vi "Distributor - Usr Ev Engine.vi"(8 "error in (no error)":errorcluster, 11 "Action":T3=enum."Get Refs") -> (0 "error out":errorcluster, 1 "Events Array":string[](array[string]), 2 "Usr Ev Refs":T2, 3 "Usr Ev Reg - Refs - cluster":T1)   [LabVIEW 2023, in "Actor_Message_Distributor.lvlib" / "Message_Distributor_Class.lvclass"]
uses:
  Message_Distributor_Class.lvclass
  Distributor - Ctrl - Action.ctl
  Distributor - Ctrl - Usr Ev Ref.ctl
  Distributor - Ctrl - Usr Ev Reg - Refs.ctl
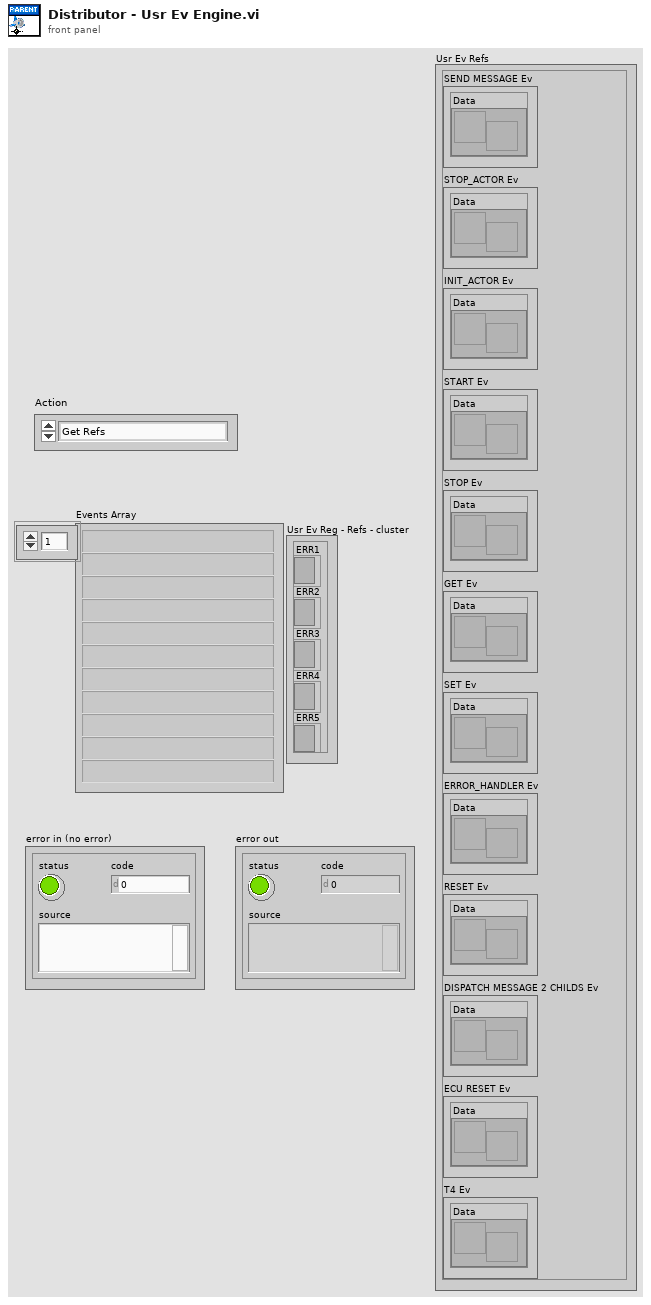
[diagram p1: front panel]
types:
  T1 = typedef "Actor_Message_Distributor.lvlib/Message_Distributor_Class.lvclass/Distributor - Ctrl - Usr Ev Reg - Refs.ctl" = cluster{"ERR1":refnum<event-registration>, "ERR2":refnum<event-registration>, "ERR3":refnum<event-registration>, "ERR4":refnum<event-registration>, "ERR5":refnum<event-registration>}
  T2 = typedef "Actor_Message_Distributor.lvlib/Message_Distributor_Class.lvclass/Distributor - Ctrl - Usr Ev Ref.ctl" = cluster{"SEND MESSAGE Ev":cluster{"Data":refnum<user-event>}, "STOP_ACTOR Ev":cluster{"Data":refnum<user-event>}, "INIT_ACTOR Ev":cluster{"Data":refnum<user-event>}, "START Ev":cluster{"Data":refnum<user-event>}, "STOP Ev":cluster{"Data":refnum<user-event>}, "GET Ev":cluster{"Data":refnum<user-event>}, "SET Ev":cluster{"Data":refnum<user-event>}, "ERROR_HANDLER Ev":cluster{"Data":refnum<user-event>}, "RESET Ev":cluster{"Data":refnum<user-event>}, "DISPATCH MESSAGE 2 CHILDS Ev":cluster{"Data":refnum<user-event>}, "ECU RESET Ev":cluster{"Data":refnum<user-event>}, "T4 Ev":cluster{"Data":refnum<user-event>}}
  T3 = typedef "Actor_Message_Distributor.lvlib/Message_Distributor_Class.lvclass/Distributor - Ctrl - Action.ctl" = enum16{"Reg Ev", "Get Refs", "Close Ev", "Populate Enum with Events"}
  T4 = enum32{"Invalid", "Standard", "Closed", "Hidden", "Minimized", "Maximized"}
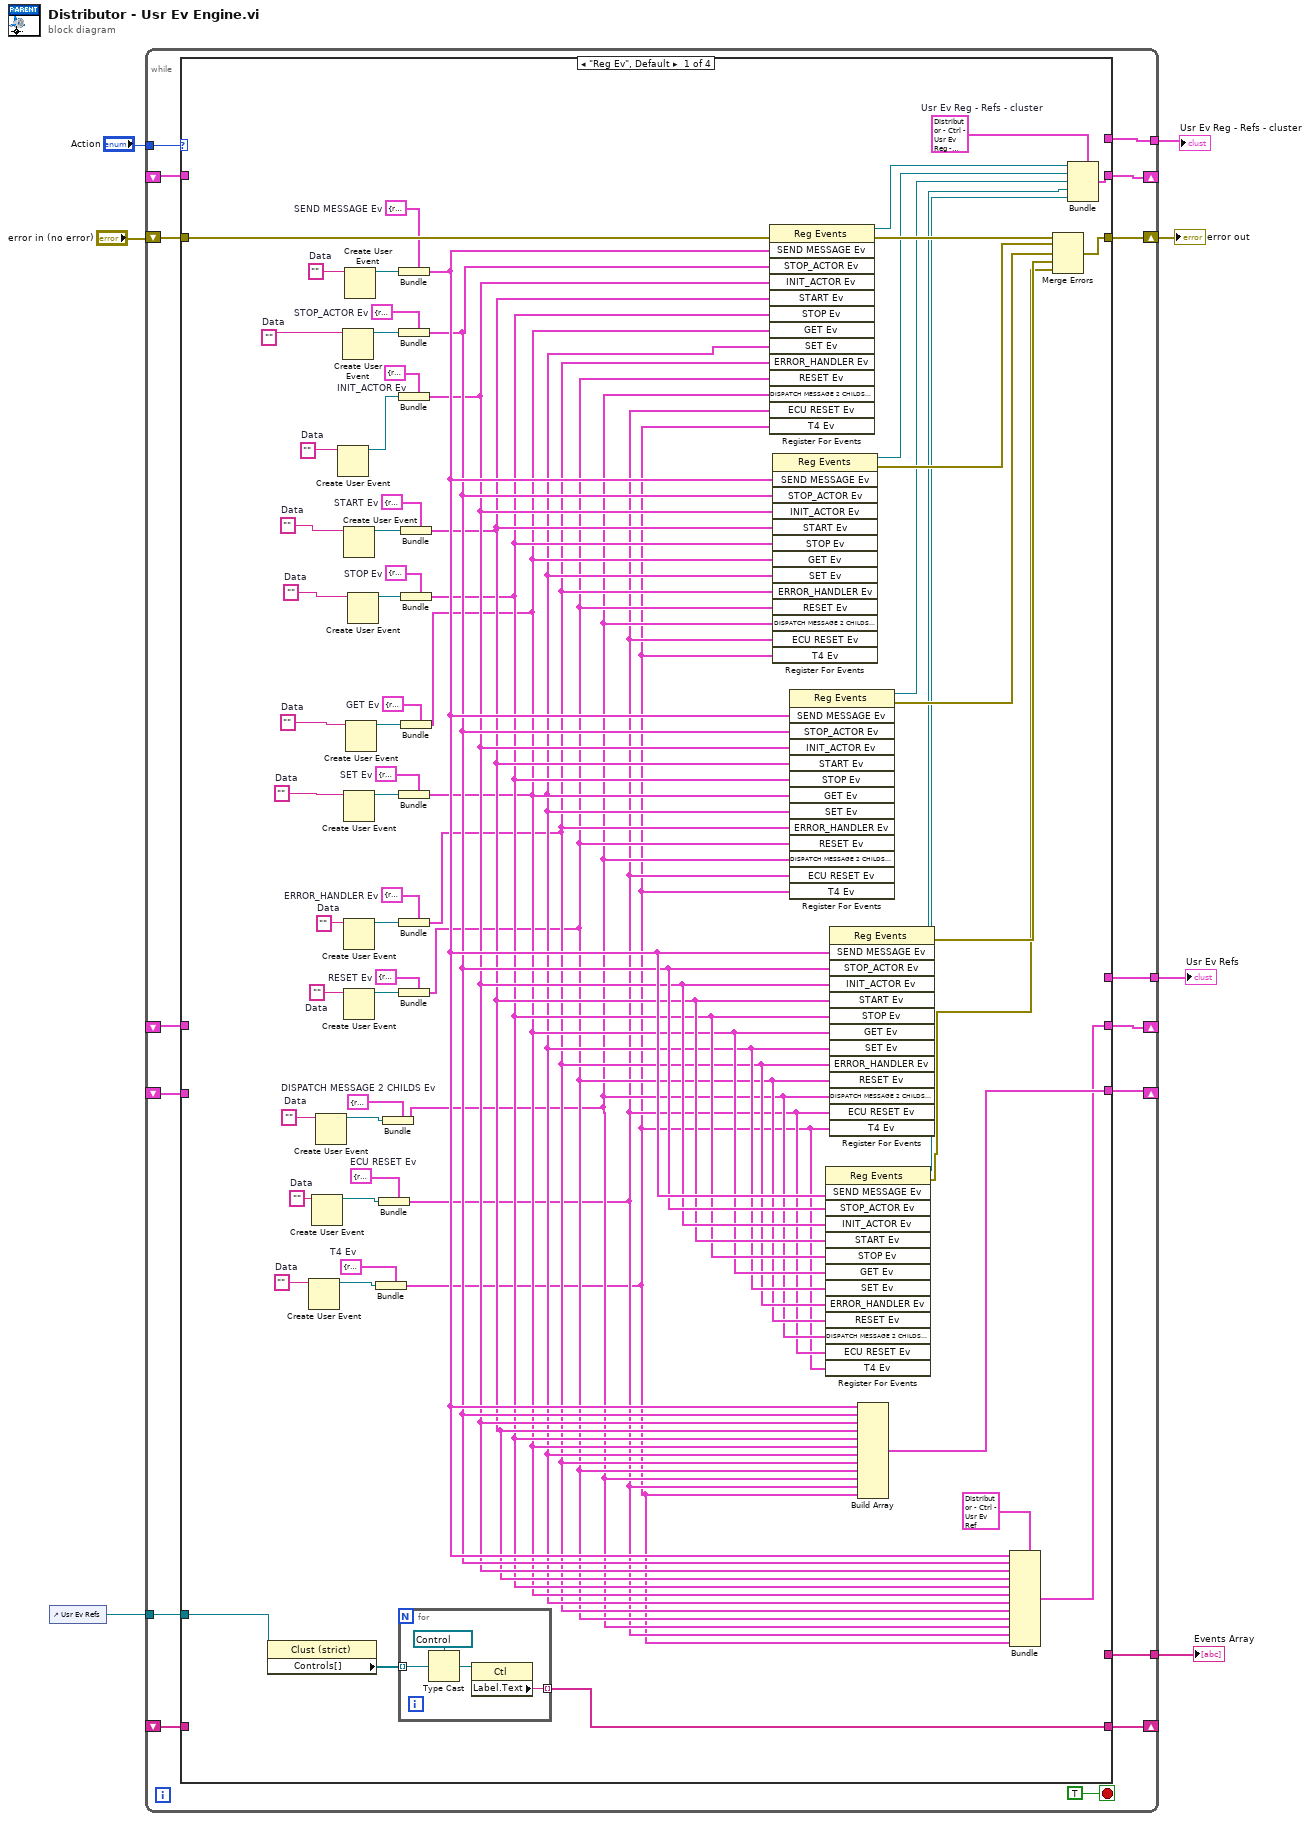
[diagram p0: block diagram]
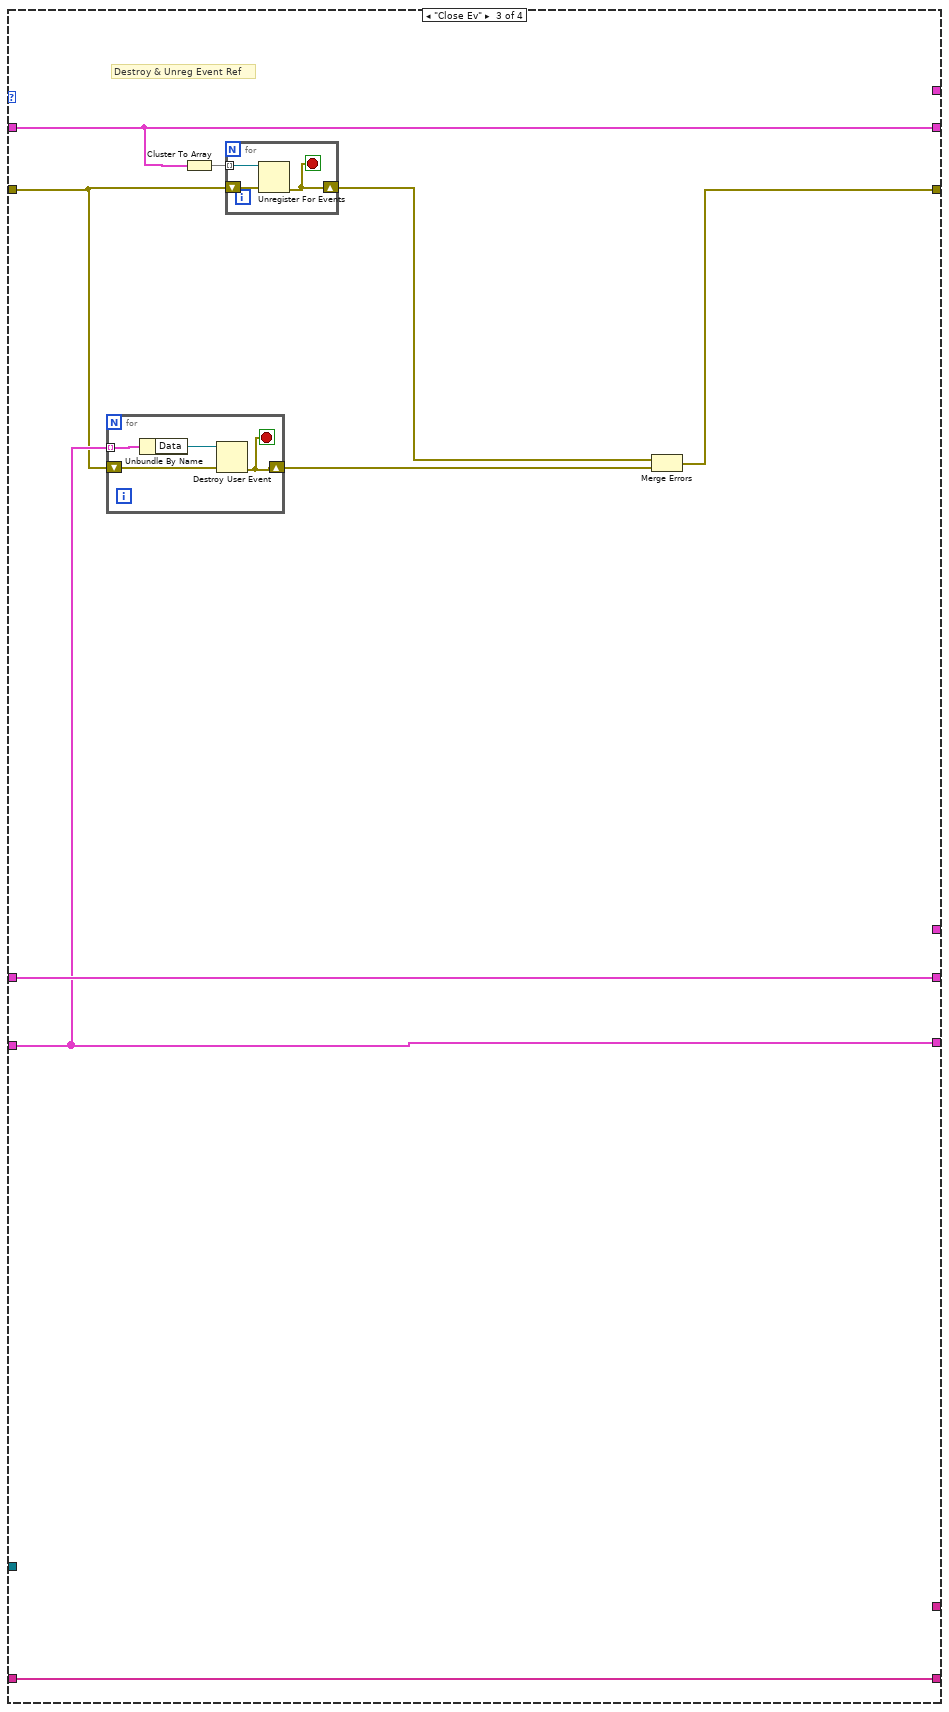
[diagram p3: hidden frame]
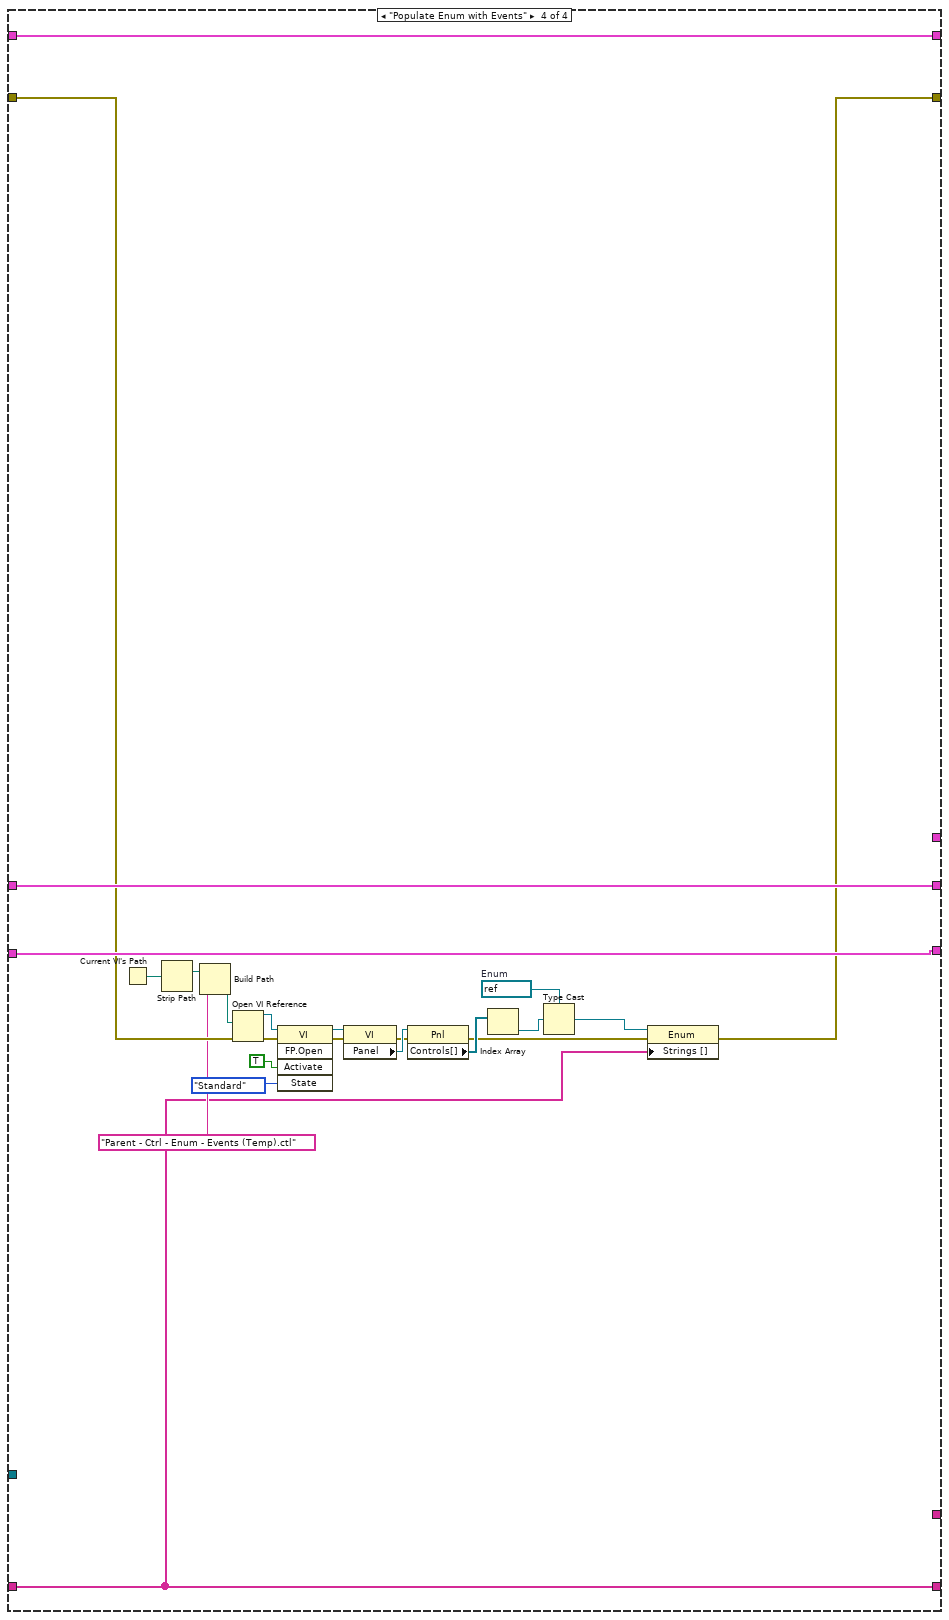
[diagram p4: hidden frame]
diagram:
  n1 = control-ref of="Usr Ev Refs"() -> (w3:refnum<vi>)
  n2 = while {
    tunnel: "Action" -> [w19]
    shift-right: [w18] -> _
    shift-left: _ -> [w17]
    shift-right: [w13] -> _
    shift-left: _ -> [w16]
    shift-right: [w21] -> _
    shift-left: _ -> [w15]
    shift-right: [w23] -> w5
    shift-left: "error in (no error)" -> [w22]
    tunnel: [w14] -> w4
    shift-right: [w11] -> _
    shift-left: _ -> [w12]
    tunnel: w3 -> [w10]
    tunnel: [w9] -> w2
    tunnel: [w8] -> w1
    stop <- TRUE stop-if-true
    n3 = case shown="\"Reg Ev\", Default" w19 {
      tunnel: [w87 w100 w108 w124] -> w23
      tunnel: w22 -> [w86 w100 w103 w125]
      tunnel: [w84 w99 w105 w123] -> w21
      tunnel: [w78 w96 w107 w139] -> w18
      tunnel: w17 -> [_ w96 w107 w139]
      tunnel: w16 -> [_ w98 w106 w138]
      tunnel: w15 -> [_ w99 w105 w123]
      tunnel: [_ w99 _ _] -> w14
      tunnel: [w79 w98 w106 w138] -> w13
      tunnel: w12 -> [_ w97 w101 w117]
      tunnel: [w76 w97 w101 w117] -> w11
      tunnel: w10 -> [w75 _ _ _]
      tunnel: [_ w97 _ _] -> w9
      tunnel: [_ w96 _ _] -> w8
      frame "Reg Ev", Default {
        w47 = cluster{"Data":refnum<user-event>} {"Data"=refnum}  # T4 Ev
        w48 = ""  # Data
        w50 = cluster{"Data":refnum<user-event>} {"Data"=refnum}  # ECU RESET Ev
        w49 = ""  # Data
        w53 = cluster{"Data":refnum<user-event>} {"Data"=refnum}  # DISPATCH MESSAGE 2 CHILDS Ev
        w54 = ""  # Data
        w56 = cluster{"Data":refnum<user-event>} {"Data"=refnum}  # RESET Ev
        w58 = cluster{"Data":refnum<user-event>} {"Data"=refnum}  # ERROR_HANDLER Ev
        w59 = cluster{"Data":refnum<user-event>} {"Data"=refnum}  # SET Ev
        w60 = cluster{"Data":refnum<user-event>} {"Data"=refnum}  # GET Ev
        w61 = cluster{"Data":refnum<user-event>} {"Data"=refnum}  # STOP Ev
        w62 = cluster{"Data":refnum<user-event>} {"Data"=refnum}  # START Ev
        w63 = cluster{"Data":refnum<user-event>} {"Data"=refnum}  # INIT_ACTOR Ev
        w64 = cluster{"Data":refnum<user-event>} {"Data"=refnum}  # STOP_ACTOR Ev
        w65 = cluster{"Data":refnum<user-event>} {"Data"=refnum}  # SEND MESSAGE Ev
        w66 = ""  # Data
        w67 = ""  # Data
        w68 = ""  # Data
        w69 = ""  # Data
        w70 = ""  # Data
        w71 = ""  # Data
        w72 = ""  # Data
        w73 = ""  # Data
        w74 = ""  # Data
        w24 = T1 {"ERR1"=refnum, "ERR2"=refnum, "ERR3"=refnum, "ERR4"=refnum, "ERR5"=refnum}  # Usr Ev Reg - Refs - cluster
        n4 = property class="Clust (strict)"(reference=w75) -> ("Controls[]"=w77:refnum<vi>[])  [unwired: 1 in, 2 out]
        n5 = Create User Event(user event datatype=w48) -> (user event=w46:refnum<user-event>)  [unwired: 1 in, 1 out]
        n6 = Create User Event(user event datatype=w49) -> (user event=w51:refnum<user-event>)  [unwired: 1 in, 1 out]
        n7 = Create User Event(user event datatype=w54) -> (user event=w52:refnum<user-event>)  [unwired: 1 in, 1 out]
        n8 = Create User Event(user event datatype=w72) -> (user event=w85:refnum<user-event>)  [unwired: 1 in, 1 out]
        n9 = Create User Event(user event datatype=w73) -> (user event=w90:refnum<user-event>)  [unwired: 1 in, 1 out]
        n10 = Create User Event(user event datatype=w71) -> (user event=w83:refnum<user-event>)  [unwired: 1 in, 1 out]
        n11 = Create User Event(user event datatype=w68) -> (user event=w80:refnum<user-event>)  [unwired: 1 in, 1 out]
        n12 = Create User Event(user event datatype=w67) -> (user event=w57:refnum<user-event>)  [unwired: 1 in, 1 out]
        n13 = Create User Event(user event datatype=w66) -> (user event=w55:refnum<user-event>)  [unwired: 1 in, 1 out]
        n14 = Create User Event(user event datatype=w74) -> (user event=w91:refnum<user-event>)  [unwired: 1 in, 1 out]
        n15 = Create User Event(user event datatype=w69) -> (user event=w81:refnum<user-event>)  [unwired: 1 in, 1 out]
        n16 = Create User Event(user event datatype=w70) -> (user event=w82:refnum<user-event>)  [unwired: 1 in, 1 out]
        n17 = Bundle(cluster=w47, "Data"=w46) -> (w26:cluster{"Data":refnum<user-event>})
        n18 = Bundle(cluster=w50, "Data"=w51) -> (w27:cluster{"Data":refnum<user-event>})
        n19 = Bundle(cluster=w53, "Data"=w52) -> (w28:cluster{"Data":refnum<user-event>})
        n20 = Bundle(cluster=w65, "Data"=w91) -> (w37:cluster{"Data":refnum<user-event>})
        n21 = Bundle(cluster=w64, "Data"=w90) -> (w36:cluster{"Data":refnum<user-event>})
        n22 = Bundle(cluster=w63, "Data"=w85) -> (w35:cluster{"Data":refnum<user-event>})
        n23 = Bundle(cluster=w59, "Data"=w80) -> (w31:cluster{"Data":refnum<user-event>})
        n24 = Bundle(cluster=w58, "Data"=w57) -> (w30:cluster{"Data":refnum<user-event>})
        n25 = Bundle(cluster=w56, "Data"=w55) -> (w29:cluster{"Data":refnum<user-event>})
        n26 = for {
          tunnel: w77 -> [w95] mode=indexing
          tunnel: [w92] -> w76 mode=indexing
          n27 = Type Cast(type=refnum<vi> refnum ("Ctl Refnum"), x=w95) -> (*(type *) &x=w93:refnum<vi>)
          n28 = property class="Ctl"(reference=w93) -> ("Label.Text"=w92:string)  [unwired: 1 in, 2 out]
        }
        n29 = Bundle(cluster=w62, "Data"=w83) -> (w34:cluster{"Data":refnum<user-event>})
        n30 = Bundle(cluster=w61, "Data"=w82) -> (w33:cluster{"Data":refnum<user-event>})
        n31 = Bundle(cluster=w60, "Data"=w81) -> (w32:cluster{"Data":refnum<user-event>})
        n32 = register-events(error in=w86, w37, w36, w35, w34, w33, w32, w31, w30, w29, w28, w27, w26) -> (reference out=w42:refnum<event-registration>, error out=w89:errorcluster)  [unwired: 1 in]
        n33 = register-events(w37, w36, w35, w34, w33, w32, w31, w30, w29, w28, w27, w26) -> (reference out=w41:refnum<event-registration>, error out=w88:errorcluster)  [unwired: 2 in]
        n34 = register-events(w37, w36, w35, w34, w33, w32, w31, w30, w29, w28, w27, w26) -> (reference out=w40:refnum<event-registration>, error out=w45:errorcluster)  [unwired: 2 in]
        n35 = register-events(w37, w36, w35, w34, w33, w32, w31, w30, w29, w28, w27, w26) -> (reference out=w38:refnum<event-registration>, error out=w43:errorcluster)  [unwired: 2 in]
        n36 = register-events(w37, w36, w35, w34, w33, w32, w31, w30, w29, w28, w27, w26) -> (reference out=w39:refnum<event-registration>, error out=w44:errorcluster)  [unwired: 2 in]
        n37 = Build Array(w37, w36, w35, w34, w33, w32, w31, w30, w29, w28, w27, w26) -> (w79:cluster{"Data":refnum<user-event>}[])
        n38 = Bundle(cluster=T2 {"SEND MESSAGE Ev"={"Data"=refnum}, "STOP_ACTOR Ev"={"Data"=refnum}, "INIT_ACTOR Ev"={"Data"=refnum}, "START Ev"={"Data"=refnum}, "STOP Ev"={"Data"=refnum}, "GET Ev"={"Data"=refnum}, "SET Ev"={"Data"=refnum}, "ERROR_HANDLER Ev"={"Data"=refnum}, "RESET Ev"={"Data"=refnum}, "DISPATCH MESSAGE 2 CHILDS Ev"={"Data"=refnum}, "ECU RESET Ev"={"Data"=refnum}, "T4 Ev"={"Data"=refnum}} ("Usr Ev Refs"), "SEND MESSAGE Ev"=w37, "STOP_ACTOR Ev"=w36, "INIT_ACTOR Ev"=w35, "START Ev"=w34, "STOP Ev"=w33, "GET Ev"=w32, "SET Ev"=w31, "ERROR_HANDLER Ev"=w30, "RESET Ev"=w29, "DISPATCH MESSAGE 2 CHILDS Ev"=w28, "ECU RESET Ev"=w27, "T4 Ev"=w26) -> (w78:T2)
        n39 = Merge Errors(w89, w88, w45, w44, w43) -> (w87:errorcluster)
        n40 = Bundle(cluster=w24, "ERR1"=w42, "ERR2"=w41, "ERR3"=w40, "ERR4"=w39, "ERR5"=w38) -> (w84:T1)
      }
      frame "Get Refs" {
      }
      frame "Close Ev" {
        # "Destroy & Unreg Event Ref"
        n41 = for {
          tunnel: w106 -> [w114] mode=indexing
          shift-right: [w115] -> w109
          shift-left: w103 -> [w116]
          stop <- w115 stop-if-true
          n42 = Unbundle By Name(w114) -> ("Data"=w113:refnum<user-event>)
          n43 = Destroy User Event(user event=w113, error in=w116) -> (error out=w115:errorcluster)
        }
        n44 = Cluster To Array(cluster=w105) -> (array=w104:refnum<event-registration>[])
        n45 = for {
          tunnel: w104 -> [w112] mode=indexing
          shift-right: [w110] -> w102
          shift-left: w103 -> [w111]
          stop <- w110 stop-if-true
          n46 = Unregister For Events(event registration refnum=w112, error in=w111) -> (error out=w110:errorcluster)
        }
        n47 = Merge Errors(w102, w109) -> (w108:errorcluster)
      }
      frame "Populate Enum with Events" {
        w134 = refnum<vi> refnum  # Enum
        n48 = Current VI's Path() -> (path=w122:path)
        n49 = Strip Path(path=w122) -> (stripped path=w120:path)  [unwired: 1 out]
        n50 = Build Path(base path=w120, name or relative path="Parent - Ctrl - Enum - Events (Temp).ctl") -> (appended path=w119:path)
        n51 = Open VI Reference(vi path=w119, error in (no error)=w125) -> (vi reference=w126:refnum<vi>, error out=w131:errorcluster)  [unwired: 4 in]
        n52 = invoke class="VI" method="FP.Open"(reference=w126, error in=w131, "Activate"=TRUE ("Activate?"), "State"=T4."Standard") -> (reference out=w127:refnum<vi>, error out=w128:errorcluster)  [unwired: 1 in, 3 out]
        n53 = property class="VI"(reference=w127, error in=w128) -> (error out=w133:errorcluster, "Panel"=w137:refnum<vi>)  [unwired: 1 out]
        n54 = property class="Pnl"(reference=w137, error in=w133) -> (error out=w132:errorcluster, "Controls[]"=w136:refnum<vi>[])  [unwired: 1 out]
        n55 = Index Array(array=w136) -> (element=w135:refnum<vi>)  [unwired: 1 in]
        n56 = Type Cast(type=w134, x=w135) -> (*(type *) &x=w118:refnum<vi>)
        n57 = property class="Enum"(reference=w118, error in=w132, "Strings []"=w117) -> (error out=w124:errorcluster)  [unwired: 1 out]
      }
    }
  }
  "error out" <- w5
  "Usr Ev Refs" <- w1
  "Usr Ev Reg - Refs - cluster" <- w4
  "Events Array" <- w2
